vi "5p1_HW_Task1_pipoat.vi"() -> ()   [LabVIEW 2016]
uses:
  <vilib>/express/express arith-compare/Formula/XNode/ExpressFormulaBlockNode.xnode
panel:
  out "Repel?":string
  out "Force (N)":dbl
  in  "Distance (m)":dbl
  in  "Q2 (C)":dbl
  in  "Q1 (C)":dbl
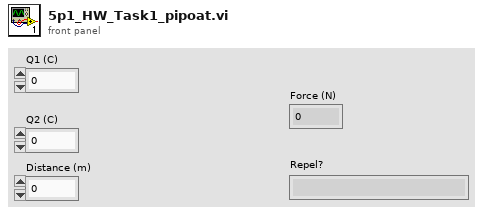
[diagram p1: front panel]
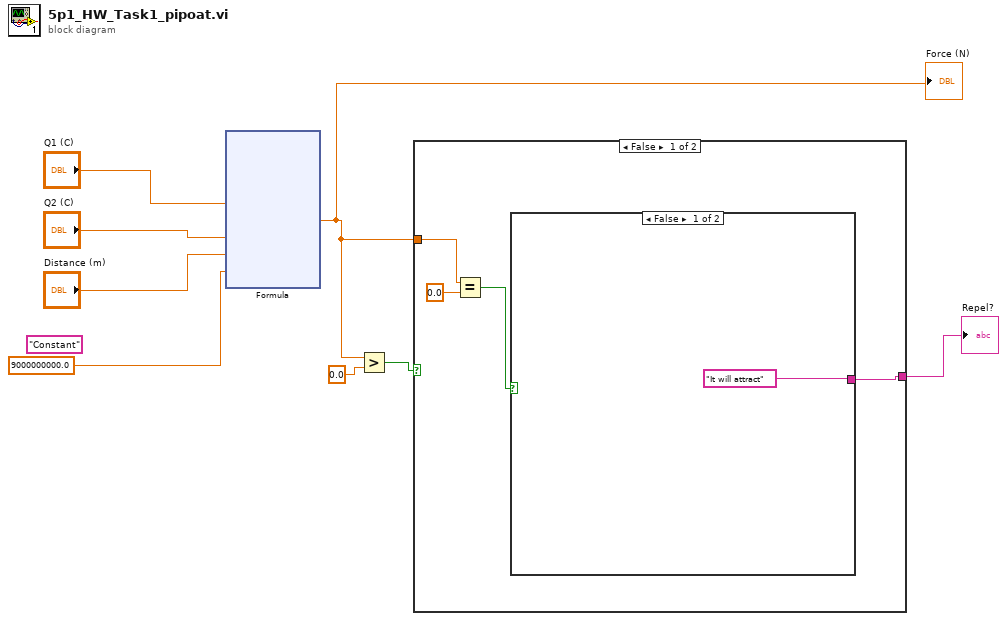
[diagram p0: block diagram]
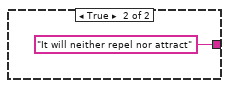
[diagram p2: hidden frame]
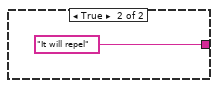
[diagram p3: hidden frame]
diagram:
  (unwired) "Constant"
  n1 = xnode "Formula"("Q1"="Q1 (C)", "Q2"="Q2 (C)", "Distance"="Distance (m)", "Constant"=9000000000.0) -> ("Result"=w1:dbl)  [unwired: 1 in, 1 out]
  "Force (N)" <- w1
  n2 = Greater?(x=w1, y=0.0) -> (0:w3:bool)
  n3 = case shown="False" w3 {
    tunnel: [w9 "It will repel"] -> w2
    tunnel: w1 -> [w12 _]
    frame False {
      n4 = Equal?(x=w12, y=0.0) -> (x = y?=w10:bool)
      n5 = case shown="False" w10 {
        tunnel: ["It will attract" "It will neither repel nor attract"] -> w9
        frame False {
        }
        frame True {
        }
      }
    }
    frame True {
    }
  }
  "Repel?" <- w2
